vi "tcp client testing.vi"() -> ()   [LabVIEW 2015]
uses:
  TCP/TCP server.lvclass
  TCP client/TCP client.lvclass
  connection/connection maintainer.lvclass
  message/communicator message.lvclass
  communicator manager/communicator manager.lvlib
  communicator/communicator.lvclass
  communicator queue/identifying queue.lvclass
  manager/queue manager.lvclass
panel:
  out "ID 5":string
  out "data 5":variant
  out "queue":refnum<class "identifying queue.lvclass">
  out "data 4":variant
  out "ID 4":string
  out "ID 3":string
  out "data 3":variant
  out "ltcp":errorcluster
  out "lerror":errorcluster
  in  "read":bool
  in  "close connn":bool
  in  "listen":bool
  out "error out 4":errorcluster
  out "error out":errorcluster
  in  "tcp":bool
  in  "data 2":string
  in  "ID 2":string
  in  "data":string
  in  "ID":string
  in  "stop":bool
  in  "send":bool
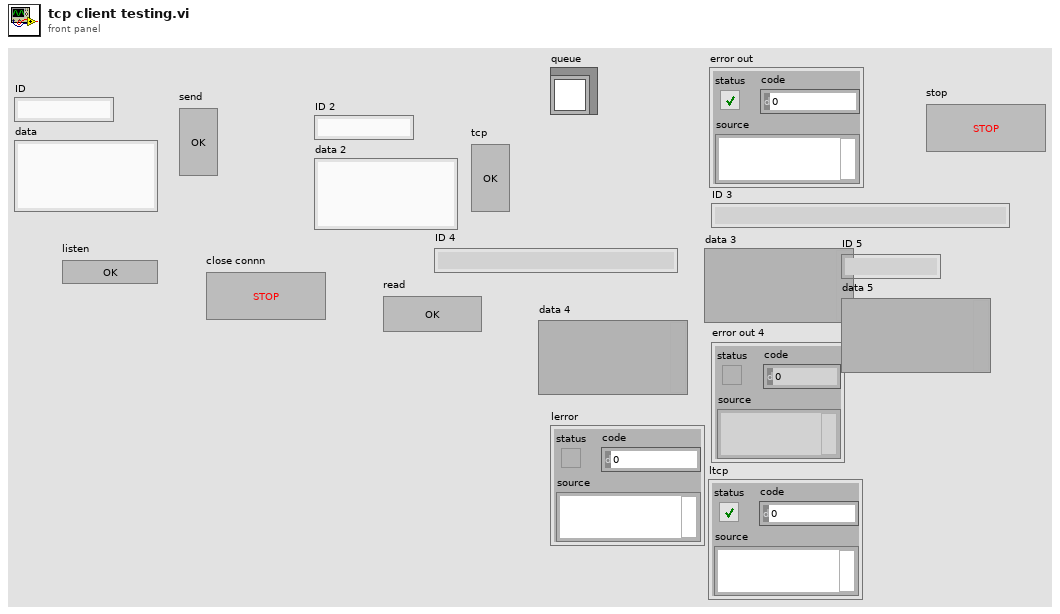
[diagram p1: front panel]
types:
  T1 = enum16{"Standard", "Buffered", "CRLF", "Immediate"}
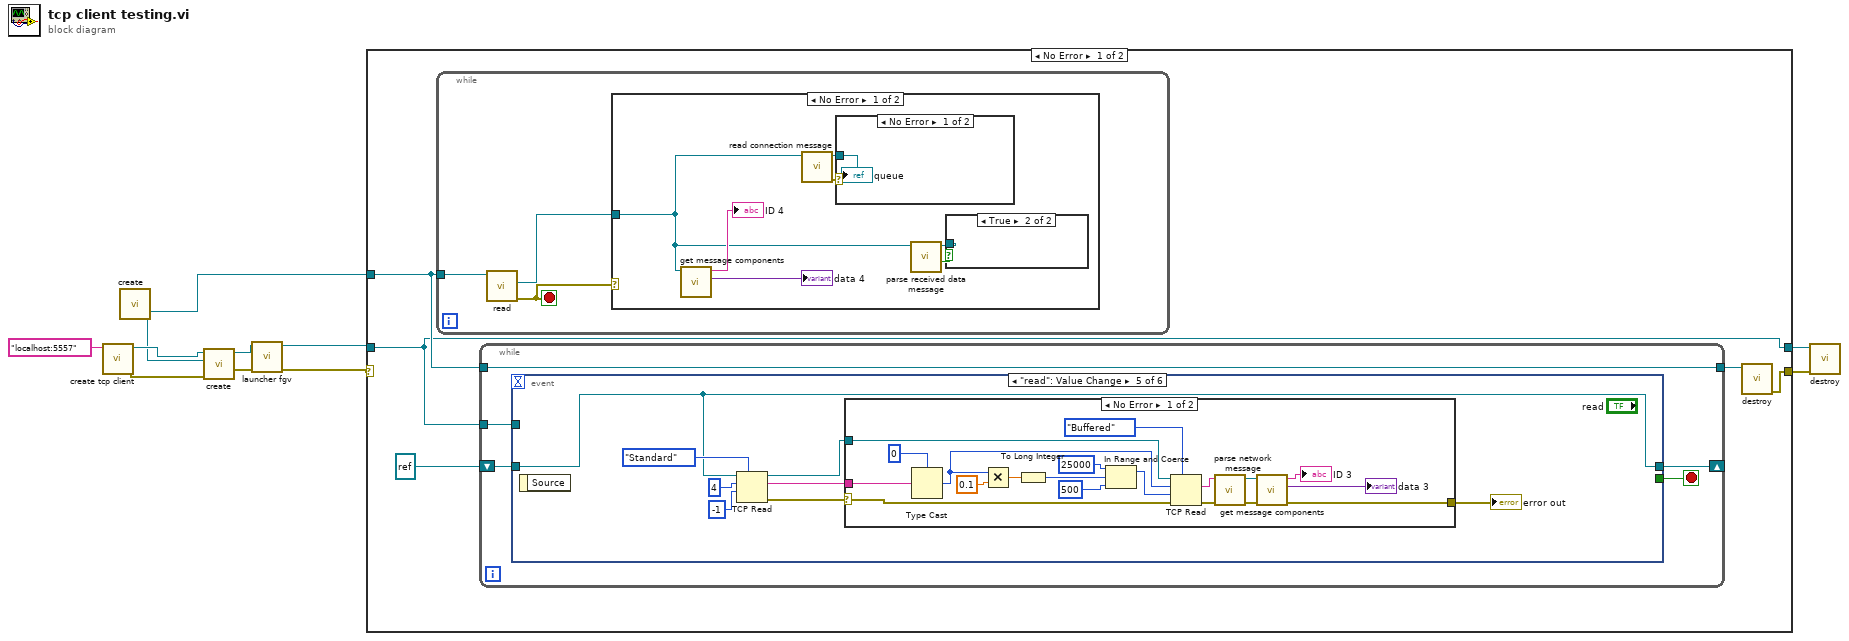
[diagram p0: block diagram]
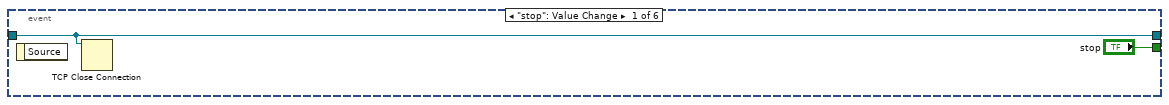
[diagram p2: hidden frame]
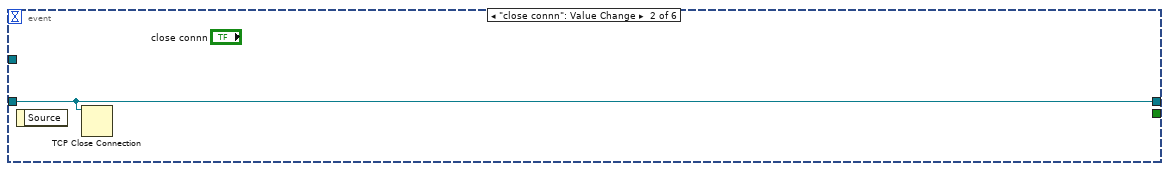
[diagram p3: hidden frame]
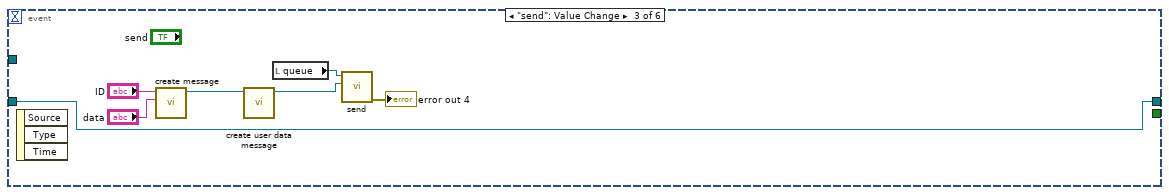
[diagram p4: hidden frame]
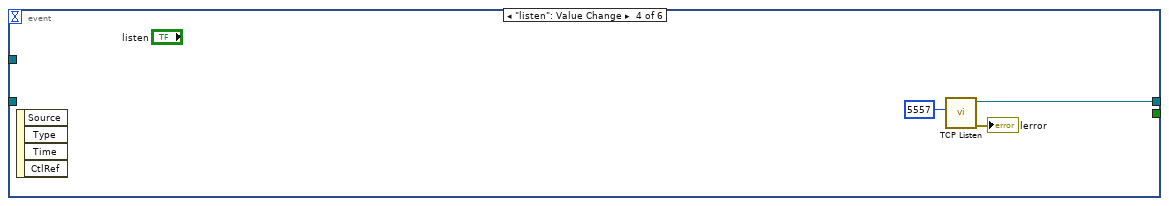
[diagram p5: hidden frame]
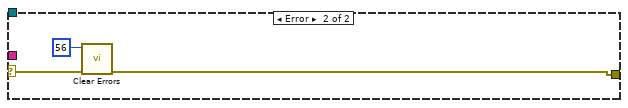
[diagram p6: hidden frame]
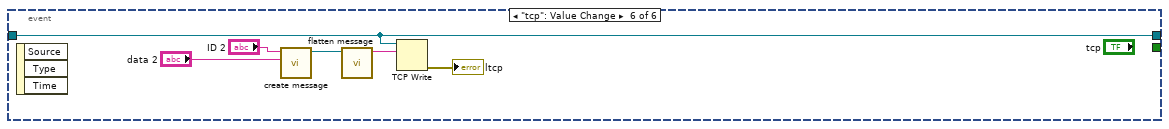
[diagram p7: hidden frame]
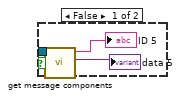
[diagram p8: hidden frame]
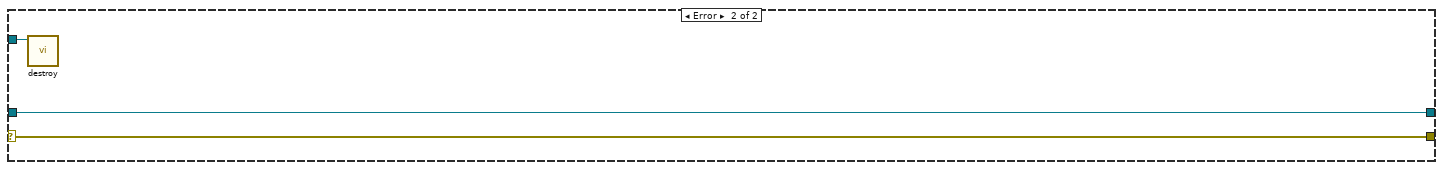
[diagram p11: hidden frame]
diagram:
  n1 = call "create tcp client.vi"("conn string"="localhost:5557" ("connection string")) -> ("error out"=w4:errorcluster, "TCP client out"=w5:refnum<class "TCP client.lvclass">)  [unwired: 9 in]
  n2 = call "create.vi"() -> ("message connection out"=w3:refnum<class "identifying queue.lvclass">)  [unwired: 10 in, 1 out]
  n3 = call "create.vi"("error in"=w4, "parent"=w3, "uninitialized communicator"=w5) -> ("error out"=w7:errorcluster, "communicator out"=w6:refnum<class "TCP client.lvclass">)  [unwired: 7 in]
  n4 = call "launcher fgv.vi"("error in"=w7, "communicator in"=w6) -> ("error out"=w1:errorcluster, "initialized communicator"=w2:refnum<class "communicator.lvclass">)  [unwired: 8 in]
  n5 = case shown="No Error" w1 {
    selector: w1 -> [_ w85]
    tunnel: [w12 w83] -> w10
    tunnel: w3 -> [w15 w84]
    tunnel: [w13 w85] -> w9
    tunnel: w2 -> [w12 w83]
    frame No Error {
      n6 = while {
        tunnel: w15 -> [w71]
        stop <- w69 stop-if-true
        n7 = call "read.vi"("identifying queue in"=w71) -> ("error out"=w69:errorcluster, "message"=w70:refnum<class "communicator message.lvclass">)  [unwired: 8 in, 1 out]
        n8 = case shown="No Error" w69 {
          tunnel: w70 -> [w72 _]
          frame No Error {
            n9 = call "get message components.vi"("message"=w72) -> ("data"=→"data 4":variant, "ID"=→"ID 4":string)  [unwired: 9 in]
            n10 = call "read connection message.vi"("communicator message in"=w72) -> ("error out"=w77:errorcluster, "queue"=w78:refnum<class "identifying queue.lvclass">)  [unwired: 9 in]
            n11 = case shown="No Error" w77 {
              tunnel: w78 -> [w82 _]
              frame No Error {
                "queue" <- w82
              }
              frame Error {
              }
            }
            n12 = call "parse received data message.vi"("message"=w72) -> ("invalid?"=w73:bool, "data"=w74:refnum<class "communicator message.lvclass">)  [unwired: 9 in]
            n13 = case shown="True" w73 {
              tunnel: w74 -> [w81 _]
              frame False {
                n14 = call "get message components.vi"("message"=w81) -> ("data"=→"data 5":variant, "ID"=→"ID 5":string)  [unwired: 9 in]
              }
              frame True {
              }
            }
          }
          frame Error {
          }
        }
      }
      n15 = while {
        tunnel: w12 -> [w18]
        tunnel: [w19] -> w14
        tunnel: w15 -> [w19]
        shift-right: [w17] -> _
        shift-left: refnum<k5> refnum ("connection ID") -> [w16]
        stop <- w20 stop-if-true
        n16 = event shown="[4] \"read\": Value Change" {
          selector: _ -> [_ _ _ _ _ _]
          dyn-events: _ -> [_ _ _ _ _ _]
          timeout: _ -> [_ _ _ _ _ _]
          tunnel: ["stop" _ _ _ _ _] -> w20
          tunnel: w18 -> [_ _ _ _ _ _]
          tunnel: [w21 w23 w28 w32 w35 w67] -> w17
          tunnel: w16 -> [w21 w23 w28 _ w35 w67]
          event "stop": Value Change {
            n17 = event-data() -> ()  [unwired: 1 in, 1 out]
            n18 = TCP Close Connection(connection ID=w21) -> ()  [unwired: 2 in, 2 out]
          }
          event "close connn": Value Change {
            n19 = event-data() -> ()  [unwired: 1 in, 1 out]
            n20 = TCP Close Connection(connection ID=w23) -> ()  [unwired: 2 in, 2 out]
          }
          event "send": Value Change {
            n21 = event-data() -> ()  [unwired: 1 in, 3 out]
            n22 = call "create message.vi"("data"="data", "ID"="ID") -> ("message"=w25:refnum<class "communicator message.lvclass">)  [unwired: 9 in]
            n23 = call "create user data message.vi"("data"=w25) -> ("message"=w24:refnum<class "communicator message.lvclass">)  [unwired: 10 in]
            n24 = local read "queue"() -> (w30:refnum<class "identifying queue.lvclass">)
            n25 = call "send.vi"("message"=w24, "message connection in"=w30) -> ("error out"=→"error out 4":errorcluster)  [unwired: 8 in, 1 out]
          }
          event "listen": Value Change {
            n26 = event-data() -> ()  [unwired: 1 in, 4 out]
            n27 = call <vilib>:"TCP Listen.vi"("port"=u16 5557) -> ("error out"=→"lerror":errorcluster, "connection ID"=w32:refnum<k5>)  [unwired: 6 in, 3 out]
          }
          event "read": Value Change {
            n28 = event-data() -> ()  [unwired: 1 in, 1 out]
            n29 = TCP Read(connection ID=w35, bytes to read=4, 7:T1."Standard" ("mode (standard)"), 9:-1 ("timeout ms (25000)")) -> (connection ID out=w36:refnum<k5>, data out=w37:string, error out=w38:errorcluster)  [unwired: 1 in]
            n30 = case shown="No Error" w38 {
              selector: w38 -> [w56 w62]
              tunnel: [w45 w60] -> w34
              tunnel: w37 -> [w59 _]
              tunnel: w36 -> [w57 _]
              frame No Error {
                n31 = Type Cast(type=0, x=w59) -> (*(type *) &x=w51:i32)
                n32 = Multiply(x=w51, y=0.1) -> (x*y=w52:dbl)
                n33 = To Long Integer(number=w52) -> (32bit integer=w47:i32)
                n34 = In Range and Coerce(upper limit=25000 ("timeout ms (25000)"), x=w47, lower limit=500 ("timeout ms (25000)")) -> (coerced(x)=w48:i32)  [unwired: 1 out]
                n35 = TCP Read(connection ID=w57, bytes to read=w51, error in (no error)=w56, 7:T1."Buffered" ("mode (standard)"), 9:w48) -> (data out=w55:string, error out=w46:errorcluster)  [unwired: 1 out]
                n36 = call "parse network message.vi"("error in"=w46, "data"=w55) -> ("error out"=w45:errorcluster, "message"=w44:refnum<class "communicator message.lvclass">)  [unwired: 8 in]
                n37 = call "get message components.vi"("message"=w44) -> ("data"=→"data 3":variant, "ID"=→"ID 3":string)  [unwired: 9 in]
              }
              frame Error {
                n38 = call <vilib>:"Clear Errors.vi"("error in (no error)"=w62, "specific error code to clear (0: all)"=56) -> ("error out"=w60:errorcluster)  [unwired: 4 in, 1 out]
              }
            }
            "error out" <- w34
          }
          event "tcp": Value Change {
            n39 = event-data() -> ()  [unwired: 1 in, 3 out]
            n40 = call "create message.vi"("data"="data 2", "ID"="ID 2") -> ("message"=w65:refnum<class "communicator message.lvclass">)  [unwired: 9 in]
            n41 = call "flatten message.vi"("data message"=w65) -> ("data"=w68:string)  [unwired: 9 in, 1 out]
            n42 = TCP Write(connection ID=w67, data in=w68) -> (error out=→"ltcp":errorcluster)  [unwired: 2 in, 2 out]
          }
        }
      }
      n43 = call "destroy.vi"("message connection in"=w14) -> ("error out"=w13:errorcluster)  [unwired: 10 in]
    }
    frame Error {
      n44 = call "destroy.vi"("message connection in"=w84) -> ()  [unwired: 10 in, 1 out]
    }
  }
  n45 = call-dynamic "destroy.vi"("error in"=w9, "communicator in"=w10) -> ()  [unwired: 9 in, 1 out]
